vi "TSLIN_LIN_Schedule_add_sort.vi"(11 "LIN Scheduling Table Array":T1[](array[typedef]) {"LIN_Transmit"."FDatas"."value 7" format="%.0x"; "LIN_Transmit"."FDatas"."value 6" format="%.0x"; "LIN_Transmit"."FDatas"."value 5" format="%.0x"; "LIN_Transmit"."FDatas"."value 4" format="%.0x"; "LIN_Transmit"."FDatas"."value 3" format="%.0x"; "LIN_Transmit"."FDatas"."value 2" format="%.0x"; "LIN_Transmit"."FDatas"."value 1" format="%.0x"; "LIN_Transmit"."FDatas"."value0" format="%.0x"; "LIN_Transmit"."Channel" items=["CHN1", "CHN2", "CHN3", "CHN4", "CHN5", "CHN6", "CHN7", "CHN8", "CHN9", "CHN10", "CHN11", "CHN12", "CHN13", "CHN14", "CHN15", "CHN16", "CHN17", "CHN18", "CHN19", "CHN20", "CHN21", "CHN22", "CHN23", "CHN24", "CHN25", "CHN26", "CHN27", "CHN28", "CHN29", "CHN30", "CHN31", "CHN32"]; "LIN_Transmit"."ID" format="%.0x"; "LIN_Transmit"."DLC" format="%.0x"; "LIN_Transmit"."Set_node_funtiontype" items=["MasterNode", "SlaveNode", "MonitorNote"]}) -> (2 "CH_array":i32[](array[numeric]), 3 "LIN Scheduling Table Array out":T1[](array[typedef]) {"LIN_Transmit"."FDatas"."value 7" format="%.0x"; "LIN_Transmit"."FDatas"."value 6" format="%.0x"; "LIN_Transmit"."FDatas"."value 5" format="%.0x"; "LIN_Transmit"."FDatas"."value 4" format="%.0x"; "LIN_Transmit"."FDatas"."value 3" format="%.0x"; "LIN_Transmit"."FDatas"."value 2" format="%.0x"; "LIN_Transmit"."FDatas"."value 1" format="%.0x"; "LIN_Transmit"."FDatas"."value0" format="%.0x"; "LIN_Transmit"."Channel" items=["CHN1", "CHN2", "CHN3", "CHN4", "CHN5", "CHN6", "CHN7", "CHN8", "CHN9", "CHN10", "CHN11", "CHN12", "CHN13", "CHN14", "CHN15", "CHN16", "CHN17", "CHN18", "CHN19", "CHN20", "CHN21", "CHN22", "CHN23", "CHN24", "CHN25", "CHN26", "CHN27", "CHN28", "CHN29", "CHN30", "CHN31", "CHN32"]; "LIN_Transmit"."ID" format="%.0x"; "LIN_Transmit"."DLC" format="%.0x"; "LIN_Transmit"."Set_node_funtiontype" items=["MasterNode", "SlaveNode", "MonitorNote"]})   [LabVIEW 2014]
uses:
  Typedef/TSLIN_Transmit.ctl
  Typedef/TSLIN_LIN Schedule_Table.ctl
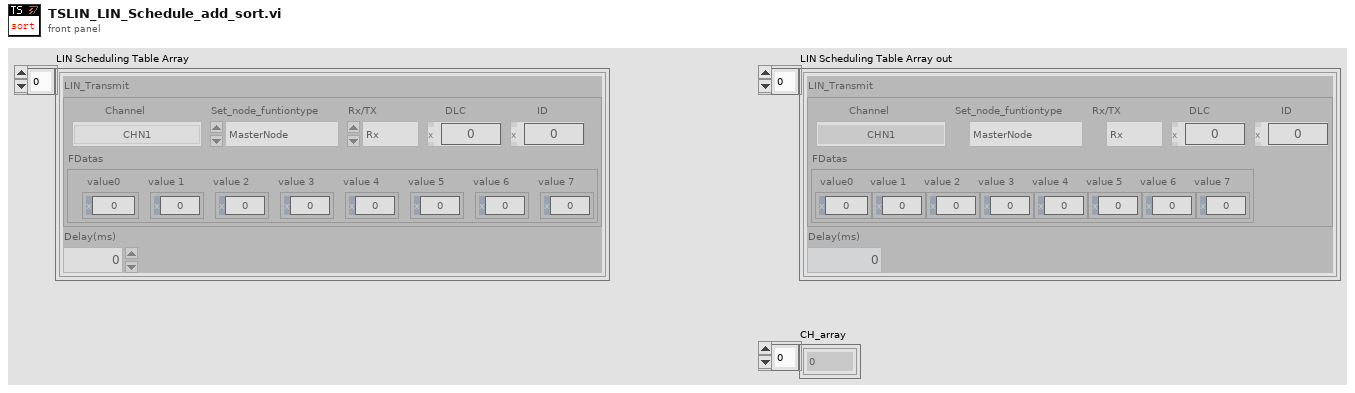
[diagram p1: front panel]
types:
  T1 = typedef "TSLIN_LIN Schedule_Table.ctl" = cluster{"LIN_Transmit":T2, "Delay(ms)":i32}
  T2 = typedef "TSLIN_Transmit.ctl" = cluster{"Channel":i32, "Rx/TX":enum16{"Rx", "Tx"}, "Set_node_funtiontype":i32, "DLC":u32, "ID":u32, "FDatas":cluster{"value0":u8, "value 1":u8, "value 2":u8, "value 3":u8, "value 4":u8, "value 5":u8, "value 6":u8, "value 7":u8}}
  T3 = cluster{"Channel":i32, "LIN scheduling table":T1}
  T4 = cluster{"Channel":i32, "LIN scheduling table":T1}[]
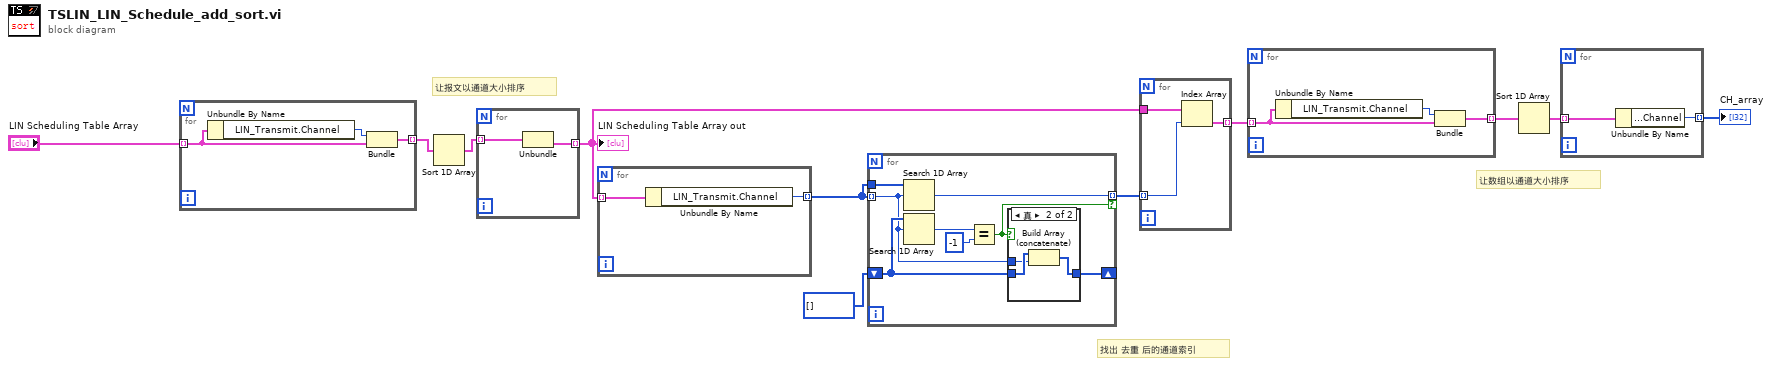
[diagram p0: block diagram]
diagram:
  # "让报文以通道大小排序"
  # "让数组以通道大小排序"
  # "找出 去重 后的通道索引"
  n1 = for {
    tunnel: "LIN Scheduling Table Array" -> [w13] mode=indexing
    tunnel: [w12] -> w2 mode=indexing
    n2 = Unbundle By Name(w13) -> ("LIN_Transmit.Channel"=w14:i32)
    n3 = Bundle("Channel"=w14, "LIN scheduling table"=w13) -> (w12:T3)  [unwired: 1 in]
  }
  n4 = Sort 1D Array(array=w2) -> (sorted array=w1:T4)
  n5 = for {
    tunnel: w1 -> [w16] mode=indexing
    tunnel: [w15] -> w10 mode=indexing
    n6 = Unbundle(w16) -> ("LIN scheduling table"=w15:T1)  [unwired: 1 out]
  }
  "LIN Scheduling Table Array out" <- w10
  n7 = for {
    tunnel: w10 -> [w18] mode=indexing
    tunnel: [w17] -> w3 mode=indexing
    n8 = Unbundle By Name(w18) -> ("LIN_Transmit.Channel"=w17:i32)
  }
  n9 = for {
    tunnel: w3 -> [w21] mode=indexing
    shift-right: [w26] -> _
    shift-left: u32[] [] -> [w25]
    tunnel: [w20] -> w5 mode=indexing if=w19
    tunnel: w3 -> [w22]
    n10 = Search 1D Array(1D array=w22, element=w21) -> (index of element=w20:i32)  [unwired: 1 in]
    n11 = Search 1D Array(1D array=w25, element=w21) -> (index of element=w23:i32)  [unwired: 1 in]
    n12 = Equal?(x=w23, y=-1) -> (x = y?=w19:bool)
    n13 = case shown="真" w19 {
      tunnel: [w27 w28] -> w26
      tunnel: w25 -> [w27 w30]
      tunnel: w21 -> [_ w29]
      frame False {
      }
      frame True {
        n14 = Build Array (concatenate)(w30, w29) -> (w28:u32[])
      }
    }
  }
  n15 = for {
    tunnel: w10 -> [w33]
    tunnel: w5 -> [w32] mode=indexing
    tunnel: [w31] -> w8 mode=indexing
    n16 = Index Array(array=w33, index=w32) -> (element=w31:T1)
  }
  n17 = for {
    tunnel: w8 -> [w35] mode=indexing
    tunnel: [w34] -> w6 mode=indexing
    n18 = Unbundle By Name(w35) -> ("LIN_Transmit.Channel"=w36:i32)
    n19 = Bundle("Channel"=w36, "LIN scheduling table"=w35) -> (w34:T3)  [unwired: 1 in]
  }
  n20 = Sort 1D Array(array=w6) -> (sorted array=w7:T4)
  n21 = for {
    tunnel: w7 -> [w38] mode=indexing
    tunnel: [w37] -> w11 mode=indexing
    n22 = Unbundle By Name(w38) -> ("LIN scheduling table.LIN_Transmit.Channel"=w37:i32)
  }
  "CH_array" <- w11
